vi "校准设置页.vi"() -> ()   [LabVIEW 2016, in "斯坦道CODMn新电路板.lvlib"]
uses:
  <vilib>/Analysis/6fits.llb/Curve Fitting Criteria.ctl
  <vilib>/Analysis/NI_AALPro.lvlib
  <vilib>/ptbypt/NI_PtbyPt.lvlib
panel:
  in  "公式切换阈值滴定数(0~9999)":dbl
  out "校准状态":T1(ring)
  out "模型刷新":bool
  in  "校准按钮":T2(radio)
  in  "校准导入":bool
  in  "曲线模型":T3={"标液浓度1"=0.0, "测量吸光度1"=0.0, "样品1启用"=FALSE, "标液浓度2"=0.0, "测量吸光度2"=0.0, "样品2启用"=FALSE, "标液浓度3"=0.0, "测量吸光度3"=0.0, "样品3启用"=FALSE, "标液浓度4"=0.0, "测量吸光度4"=0.0, "样品4启用"=FALSE, "标液浓度5"=0.0, "测量吸光度5"=0.0, "样品5启用"=FALSE, "模型"=enum."线性", "精度"=4.0, "XY图"=[], "拟合公式"="", "r^2"=0.0, "标样一校准时间"=timestamp(0 s since 1904-01-01), "标样二校准时间"=timestamp(0 s since 1904-01-01), "标样三校准时间"=timestamp(0 s since 1904-01-01), "标样四校准时间"=timestamp(0 s since 1904-01-01), "标样五校准时间"=timestamp(0 s since 1904-01-01), "二次方程"={"x^2"=0.0, "K"=0.0, "B"=0.0}, "标定时间"=timestamp(0 s since 1904-01-01)} {"标定时间" format="%<%Y/%m/%d %H:%M:%S>T"; "标样五校准时间" format="%<%Y/%m/%d %H:%M:%S>T"; "标样四校准时间" format="%<%Y/%m/%d %H:%M:%S>T"; "标样三校准时间" format="%<%Y/%m/%d %H:%M:%S>T"; "标样二校准时间" format="%<%Y/%m/%d %H:%M:%S>T"; "标样一校准时间" format="%<%Y/%m/%d %H:%M:%S>T"; "r^2" format="%.7f"; "测量吸光度5" format="%#.6f"; "测量吸光度4" format="%#.6f"; "测量吸光度3" format="%#.6f"; "测量吸光度2" format="%#.6f"; "测量吸光度1" format="%#.6f"}
  in  "测量模式":T4(ring)
  in  "参数下拉列表":u16(ring) items=["CODMn"=21]
  in  "量程下拉列表":enum16{"低量程1", "低量程2", "高量程1", "高量程2"}(ring)
  # "校准时间"
  # "标液浓度"
  # "滴定数"
  # "标液一"
  # "标液二"
  # "标液三"
  # "零点"
  # "跨度"
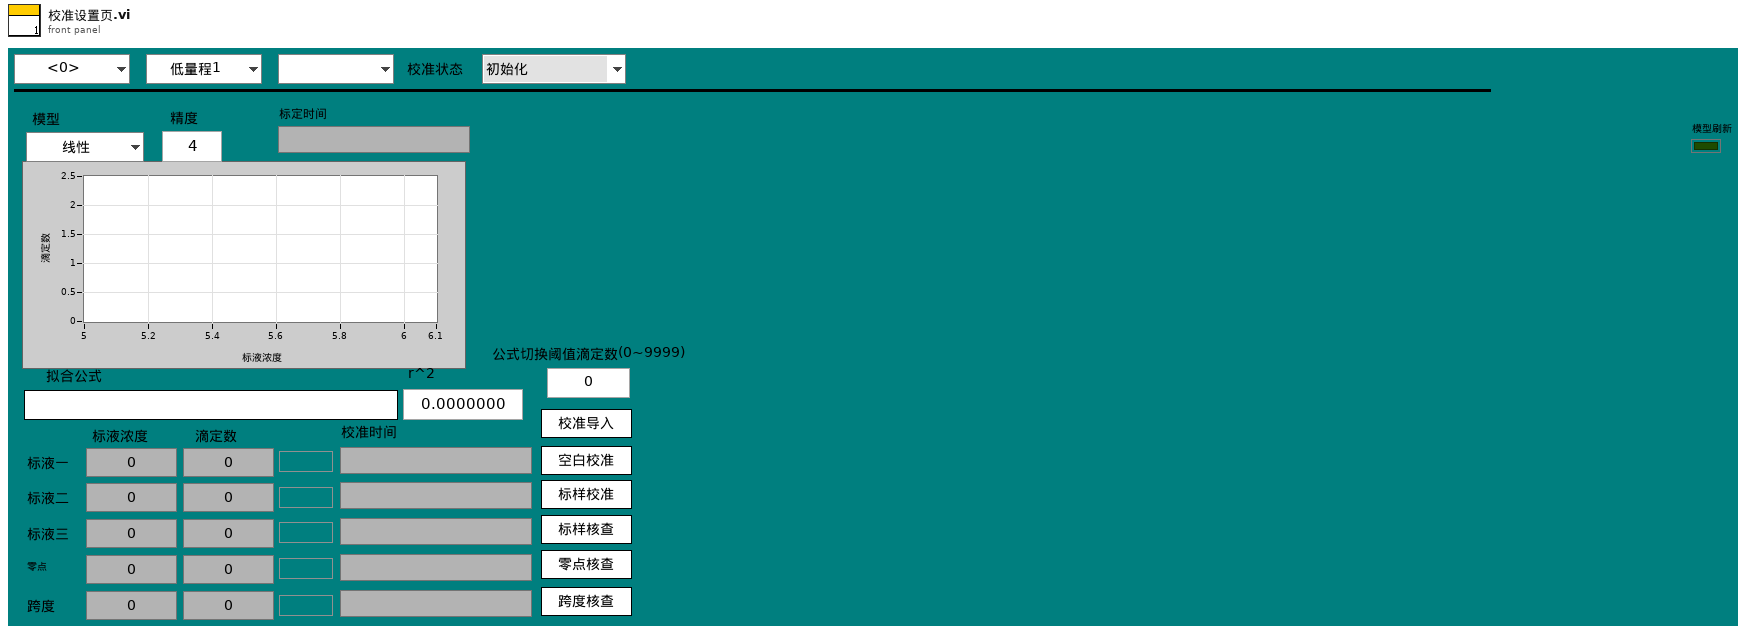
[diagram p1: front panel]
types:
  T1 = enum16{"初始化", "校准启动", "校准运行中", "测试结束", "获取校准数据", "填充校准数据", "流程结束"}
  T2 = enum32{"未选择", "空白校准", "标样校准", "标样核查", "零点核查", "跨度核查"}
  T3 = cluster{"标液浓度1":dbl, "测量吸光度1":dbl, "样品1启用":bool, "标液浓度2":dbl, "测量吸光度2":dbl, "样品2启用":bool, "标液浓度3":dbl, "测量吸光度3":dbl, "样品3启用":bool, "标液浓度4":dbl, "测量吸光度4":dbl, "样品4启用":bool, "标液浓度5":dbl, "测量吸光度5":dbl, "样品5启用":bool, "模型":enum32{"线性", "多项式"}, "精度":dbl, "XY图":cluster{"X Values":dbl[], "Y Values":dbl[]}[], "拟合公式":string, "r^2":dbl, "标样一校准时间":timestamp, "标样二校准时间":timestamp, "标样三校准时间":timestamp, "标样四校准时间":timestamp, "标样五校准时间":timestamp, "二次方程":cluster{"x^2":dbl, "K":dbl, "B":dbl}, "标定时间":timestamp}
  T4 = enum16{"", "水样测量", "标样核查", "零点核查", "跨度核查", "空白测试", "平行样测试", "加标回收"}
  T5 = enum8{"Enabled", "Disabled", "Disabled and Grayed Out"}
  T6 = cluster{"标液浓度1":dbl, "测量吸光度1":dbl, "样品1启用":bool, "标液浓度2":dbl, "测量吸光度2":dbl, "样品2启用":bool, "标液浓度3":dbl, "测量吸光度3":dbl, "样品3启用":bool, "标液浓度4":dbl, "测量吸光度4":dbl, "样品4启用":bool, "标液浓度5":dbl, "测量吸光度5":dbl, "样品5启用":bool, "模型":enum32{"线性", "多项式"}, "精度":dbl, "XY图":cluster{"X Values":dbl[], "Y Values":dbl[]}[], "拟合公式":string, "r^2":dbl, "标样一校准时间":timestamp, "标样二校准时间":timestamp, "标样三校准时间":timestamp, "标样四校准时间":timestamp, "标样五校准时间":timestamp, "二次方程":cluster{"c":dbl, "x":dbl, "x^2":dbl}, "标定时间":timestamp}[][]
  T7 = cluster{"标液浓度1":dbl, "测量吸光度1":dbl, "样品1启用":bool, "标液浓度2":dbl, "测量吸光度2":dbl, "样品2启用":bool, "标液浓度3":dbl, "测量吸光度3":dbl, "样品3启用":bool, "标液浓度4":dbl, "测量吸光度4":dbl, "样品4启用":bool, "标液浓度5":dbl, "测量吸光度5":dbl, "样品5启用":bool, "模型":enum32{"线性", "多项式"}, "精度":dbl, "XY图":cluster{"X Values":dbl[], "Y Values":dbl[]}[], "拟合公式":string, "r^2":dbl, "标样一校准时间":timestamp, "标样二校准时间":timestamp, "标样三校准时间":timestamp, "标样四校准时间":timestamp, "标样五校准时间":timestamp, "二次方程":cluster{"c":dbl, "x":dbl, "x^2":dbl}, "标定时间":timestamp}
  T8 = typedef "NI_AALPro.lvlib/Curve Fitting Criteria.ctl" = u16
  T9 = enum32{"Bad", "Idle", "Run top level", "Running"}
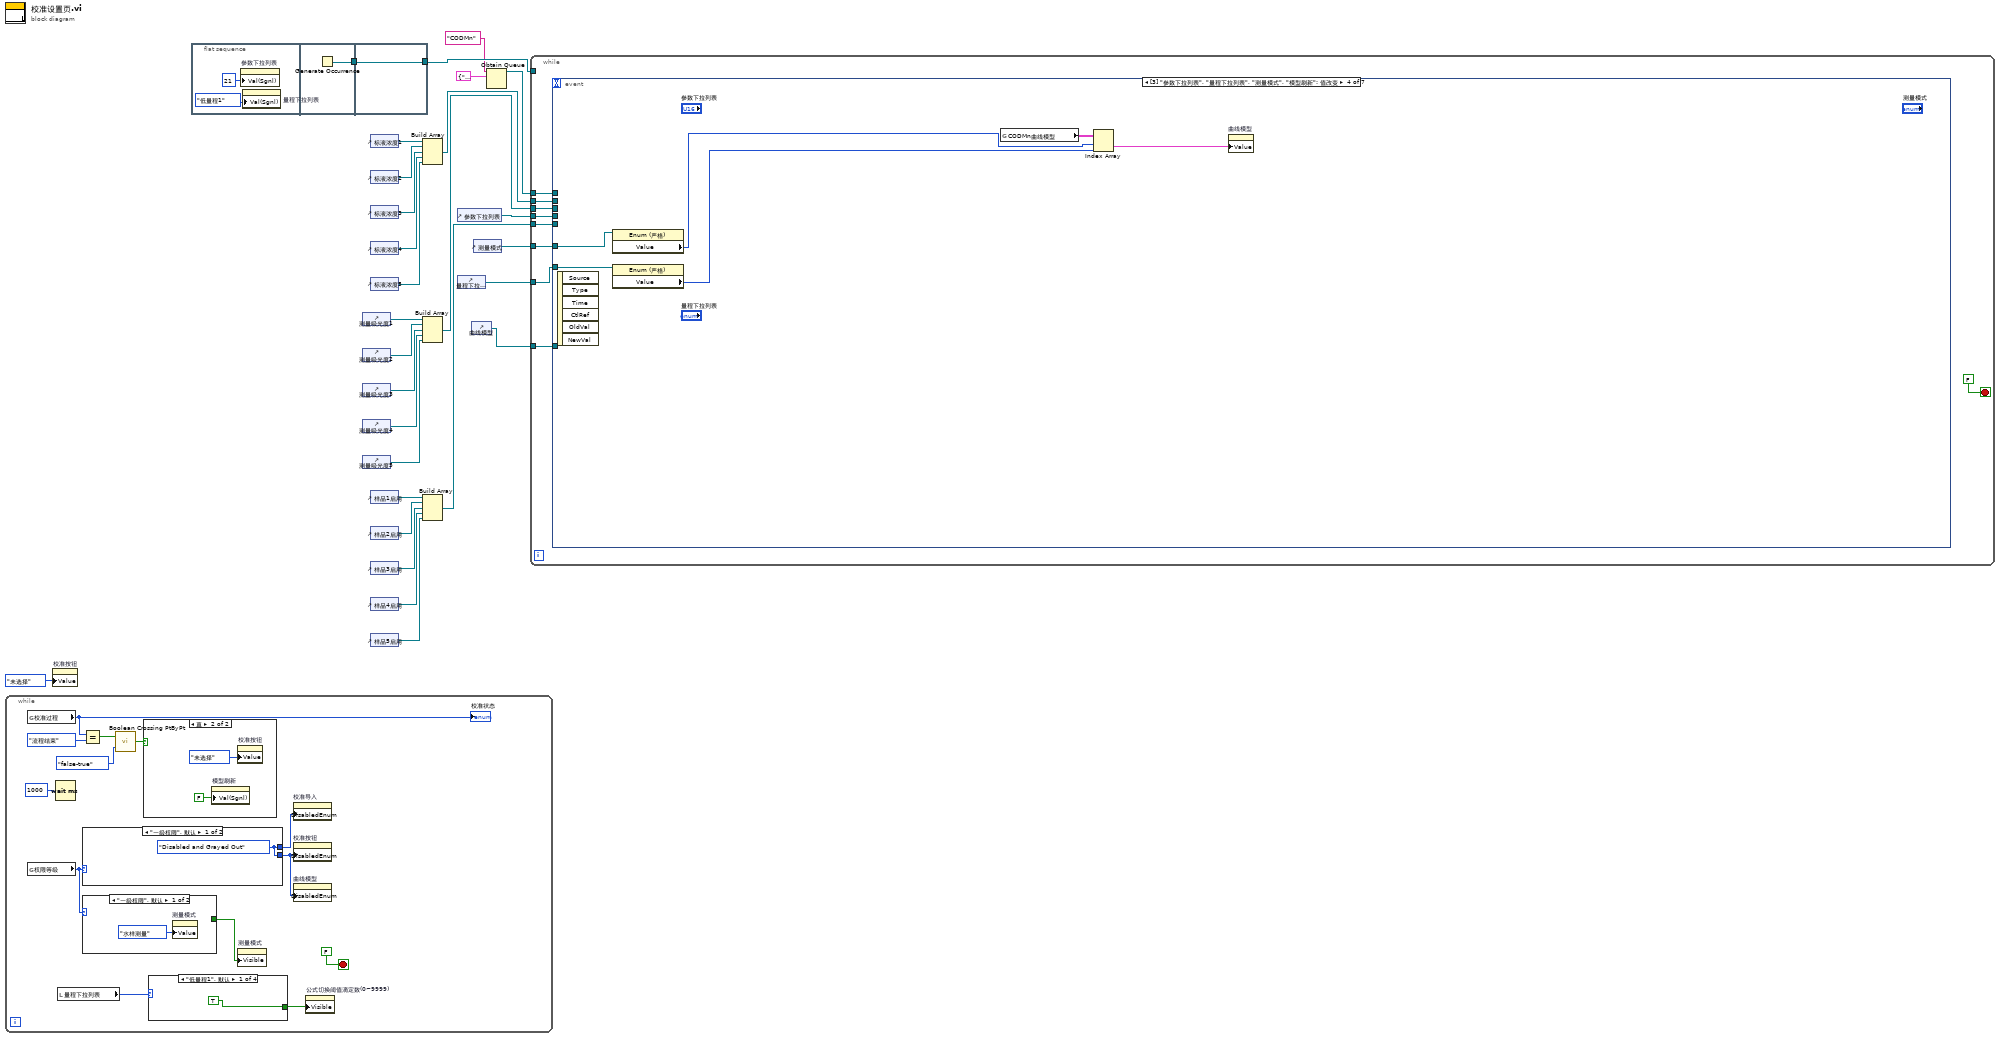
[diagram p0: block diagram]
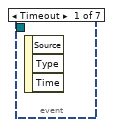
[diagram p2: hidden frame]
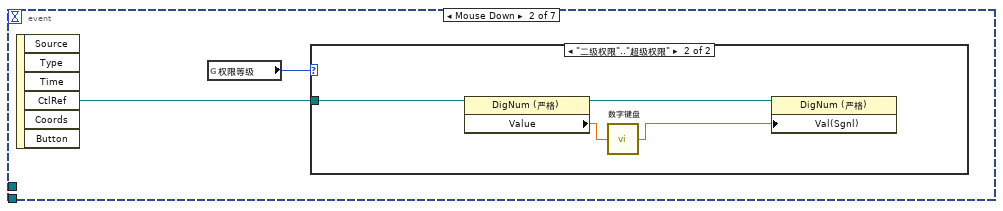
[diagram p3: hidden frame]
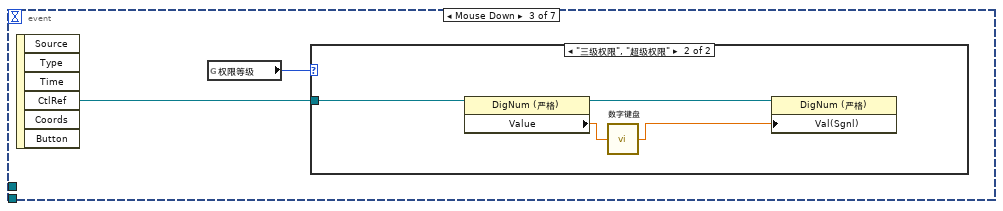
[diagram p5: hidden frame]
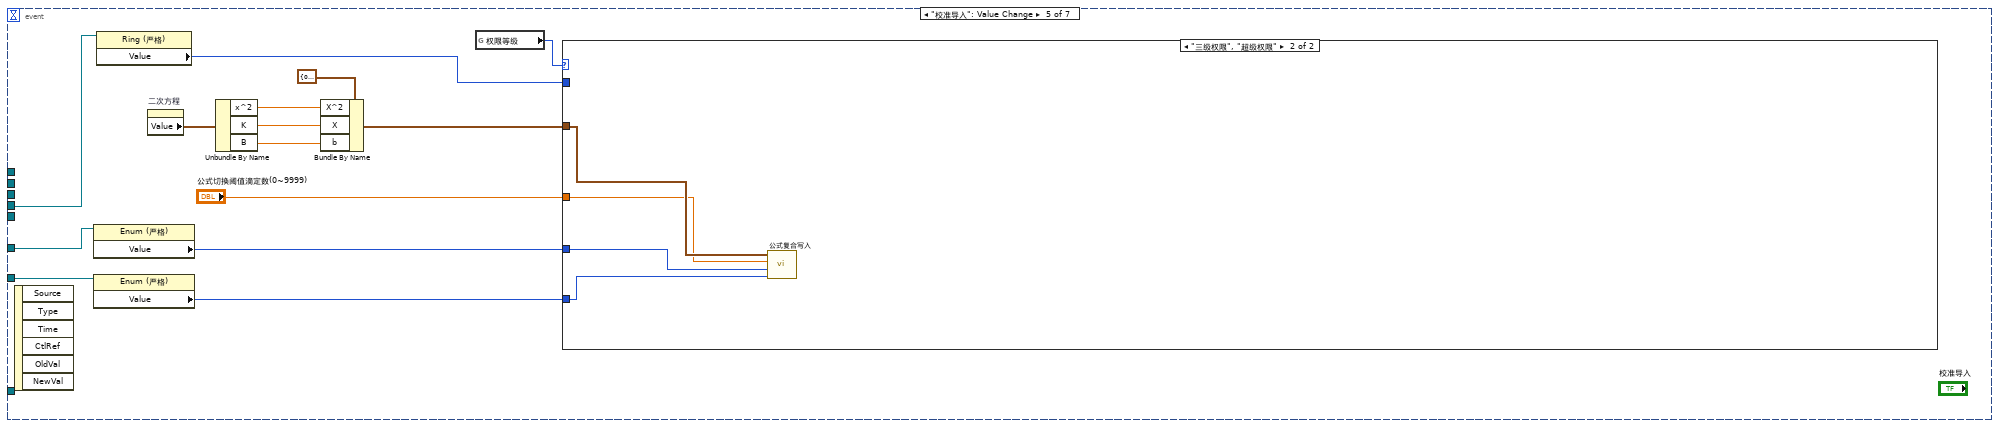
[diagram p7: hidden frame]
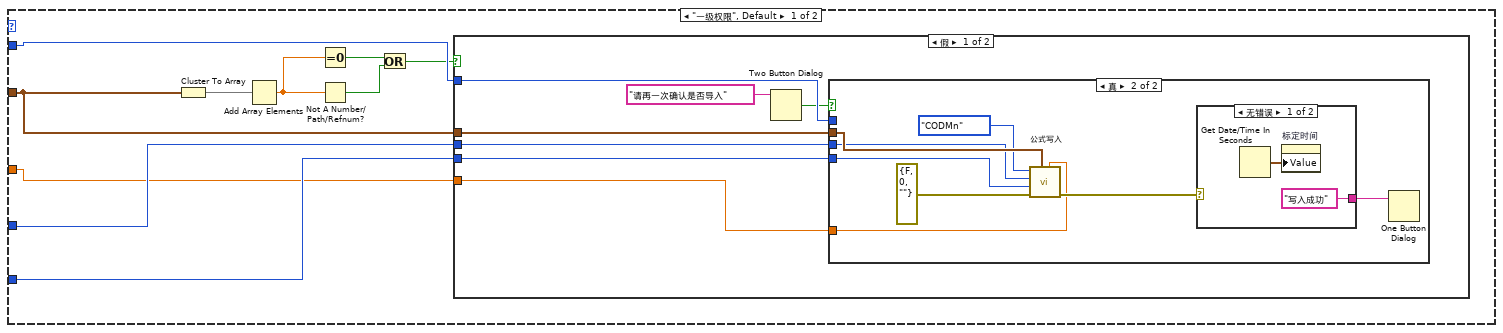
[diagram p8: hidden frame]
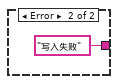
[diagram p10: hidden frame]
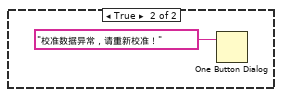
[diagram p11: hidden frame]
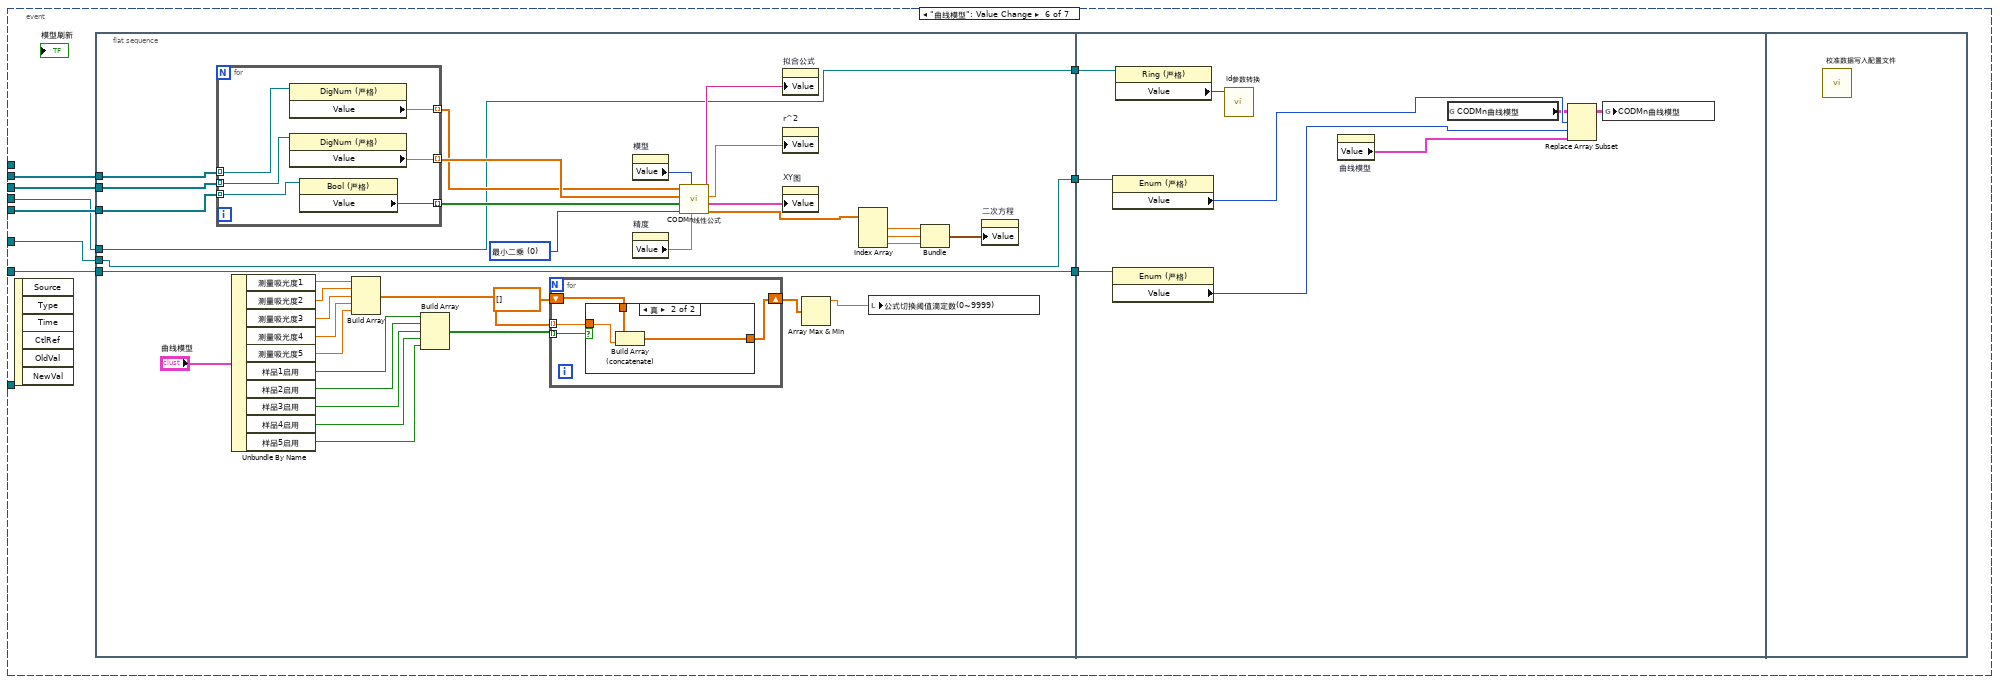
[diagram p12: hidden frame]
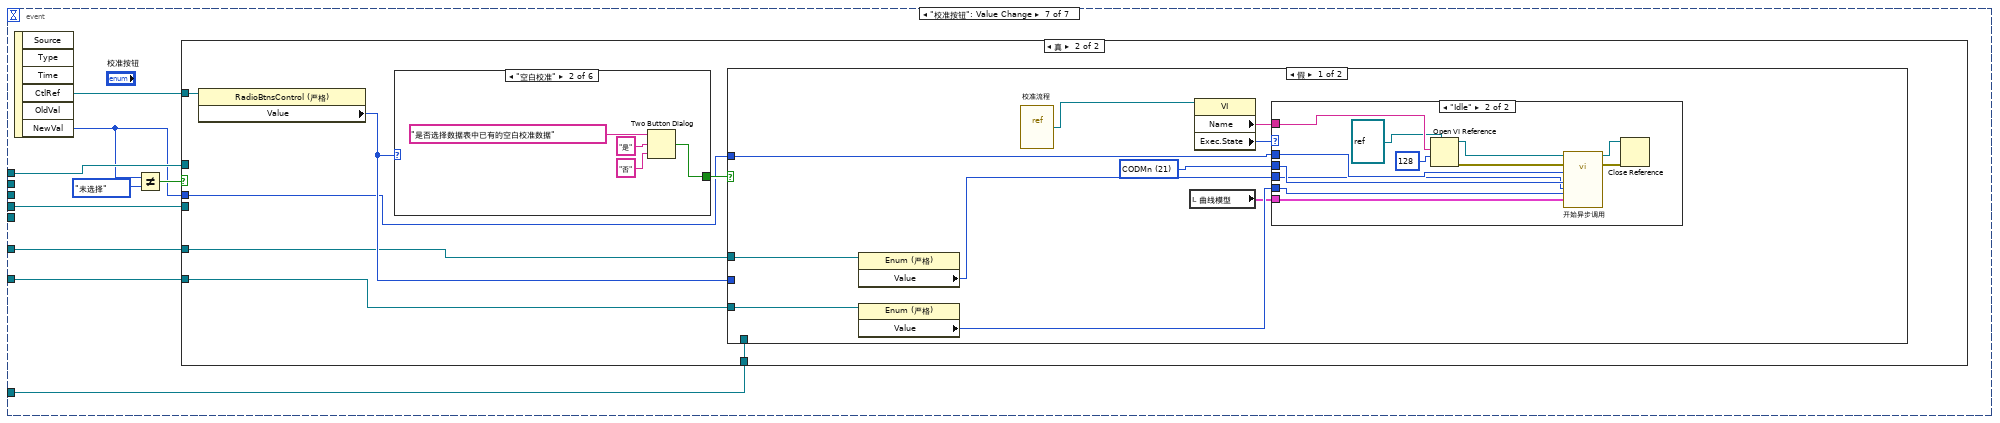
[diagram p14: hidden frame]
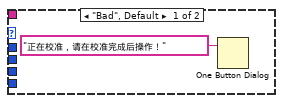
[diagram p16: hidden frame]
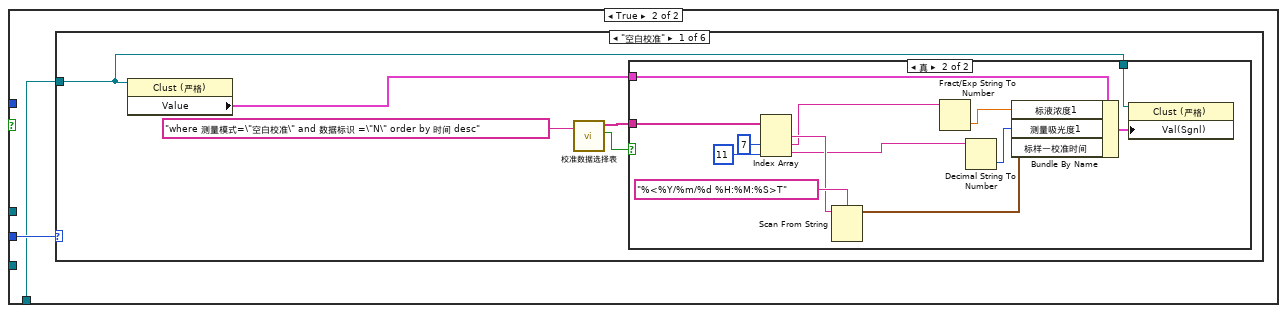
[diagram p17: hidden frame]
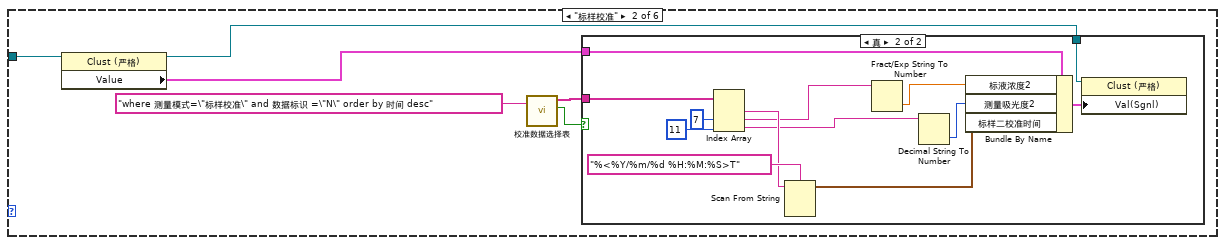
[diagram p19: hidden frame]
diagram:
  n1 = while {
    stop <- FALSE stop-if-true
    n2 = global read "VARCODMn全局变量.vi" "校准过程"() -> (w31:T1)
    "校准状态" <- w31
    n3 = global read "VARCODMn全局变量.vi" "权限等级"() -> (w38:enum16{"一级权限", "二级权限", "三级权限", "超级权限"})
    n4 = Wait (ms)(milliseconds to wait=u32 1000 ("等待时间（毫秒）")) -> ()  [unwired: 1 out]
    n5 = local read "量程下拉列表"() -> (w30:enum16{"低量程1", "低量程2", "高量程1", "高量程2"})
    n6 = case shown="\"一级权限\", 默认" w38 {
      tunnel: [w48 w49] -> w36
      tunnel: [w48 w49] -> w39
      frame "一级权限", Default {
        w48 = T5."Disabled and Grayed Out" ("禁用")
      }
      frame "二级权限".."超级权限" {
        w49 = T5."Enabled" ("禁用")
      }
    }
    n7 = case shown="\"一级权限\", 默认" w38 {
      tunnel: [_ TRUE ("可见")] -> w37
      frame "一级权限", Default {
        n8 = property on="测量模式" class="Enum (严格)"("Value"=T4."水样测量" ("测量模式")) -> ()  [unwired: 2 in, 2 out]
      }
      frame "三级权限", "超级权限" {
      }
    }
    n9 = Equal?(x=w31, y=T1."流程结束") -> (x = y?=w34:bool)
    n10 = call <vilib>:"Boolean Crossing PtByPt.vi"("direction"=enum16{"either", "false-true", "true-false"}."false-true", "input"=w34) -> ("crossing"=w32:bool)  [unwired: 1 in]
    n11 = case shown="真" w32 {
      frame False {
      }
      frame True {
        n12 = property on="模型刷新" class="Bool (严格)"("Val(Sgnl)"=FALSE ("值(信号)")) -> ()  [unwired: 2 in, 2 out]
        n13 = property on="校准按钮" class="RadioBtnsControl (严格)"("Value"=T2."未选择" ("校准按钮")) -> ()  [unwired: 2 in, 2 out]
      }
    }
    n14 = case shown="\"低量程1\", 默认" w30 {
      tunnel: [TRUE _ TRUE _] -> w29
      frame "低量程1", Default {
      }
      frame "低量程2" {
      }
      frame "高量程1" {
      }
      frame "高量程2" {
      }
    }
    n15 = property on="测量模式" class="Enum (严格)"("Visible"=w37) -> ()  [unwired: 2 in, 2 out]
    n16 = property on="校准导入" class="Bool"("DisabledEnum"=w39) -> ()  [unwired: 2 in, 2 out]
    n17 = property on="校准按钮" class="RadioBtnsControl (严格)"("DisabledEnum"=w36) -> ()  [unwired: 2 in, 2 out]
    n18 = property on="曲线模型" class="Clust (严格)"("DisabledEnum"=w36) -> ()  [unwired: 2 in, 2 out]
    n19 = property on="公式切换阈值滴定数(0~9999)" class="DigNum (严格)"("Visible"=w29) -> ()  [unwired: 2 in, 2 out]
  }
  n20 = property on="校准按钮" class="RadioBtnsControl (严格)"("Value"=T2."未选择" ("校准按钮")) -> ()  [unwired: 2 in, 2 out]
  n21 = flat-sequence {
    tunnel: [w52] -> w28
    tunnel: [w53] -> w27
    tunnel: w28 -> [w53]
    frame #0 {
      n22 = property on="参数下拉列表" class="Ring (严格)"("Val(Sgnl)"=u16 21 ("值(信号)")) -> ()  [unwired: 2 in, 2 out]
      n23 = property on="量程下拉列表" class="Enum (严格)"("Val(Sgnl)"=enum16{"低量程1", "低量程2", "高量程1", "高量程2"}."低量程1" ("值(信号)")) -> ()  [unwired: 2 in, 2 out]
    }
    frame #1 {
      n24 = Generate Occurrence() -> (w52:refnum<k4>)
    }
    frame #2 {
    }
  }
  n25 = control-ref of="测量吸光度1"() -> (w15:refnum<vi>)
  n26 = control-ref of="测量吸光度2"() -> (w16:refnum<vi>)
  n27 = control-ref of="测量吸光度3"() -> (w17:refnum<vi>)
  n28 = control-ref of="测量吸光度4"() -> (w18:refnum<vi>)
  n29 = control-ref of="测量吸光度5"() -> (w19:refnum<vi>)
  n30 = control-ref of="标液浓度1"() -> (w13:refnum<vi>)
  n31 = control-ref of="标液浓度2"() -> (w12:refnum<vi>)
  n32 = control-ref of="标液浓度3"() -> (w11:refnum<vi>)
  n33 = control-ref of="标液浓度4"() -> (w10:refnum<vi>)
  n34 = control-ref of="标液浓度5"() -> (w9:refnum<vi>)
  n35 = control-ref of="样品1启用"() -> (w25:refnum<vi>)
  n36 = control-ref of="样品2启用"() -> (w24:refnum<vi>)
  n37 = control-ref of="样品3启用"() -> (w23:refnum<vi>)
  n38 = control-ref of="样品4启用"() -> (w22:refnum<vi>)
  n39 = control-ref of="样品5启用"() -> (w21:refnum<vi>)
  n40 = Build Array(w13, w12, w11, w10, w9) -> (w8:refnum<vi>[])
  n41 = Build Array(w15, w16, w17, w18, w19) -> (w14:refnum<vi>[])
  n42 = Build Array(w25, w24, w23, w22, w21) -> (w20:refnum<vi>[])
  n43 = control-ref of="参数下拉列表"() -> (w26:refnum<vi>)
  n44 = control-ref of="量程下拉列表"() -> (w6:refnum<vi>)
  n45 = control-ref of="曲线模型"() -> (w1:refnum<vi>)
  n46 = control-ref of="测量模式"() -> (w7:refnum<vi>)
  n47 = Obtain Queue(name (unnamed)="CODMn" ("名称（未命名）"), element data type=cluster{"命令":string, "data":variant} {"命令"="", "data"=variant}) -> (queue out=w4:refnum<queue>)  [unwired: 3 in, 2 out]
  n48 = while {
    tunnel: w27 -> [_]
    tunnel: w26 -> [w61]
    tunnel: w20 -> [w60]
    tunnel: w14 -> [w59]
    tunnel: w8 -> [w58]
    tunnel: w7 -> [w57]
    tunnel: w6 -> [w56]
    tunnel: w4 -> [w55]
    tunnel: w1 -> [w54]
    stop <- FALSE stop-if-true
    n49 = event shown="[3] \"参数下拉列表\", \"量程下拉列表\", \"测量模式\", \"模型刷新\": 值改变" {
      selector: _ -> [_ _ _ _ _ _ _]
      dyn-events: _ -> [_ _ _ _ _ _ _]
      timeout: _ -> [_ _ _ _ _ _ _]
      tunnel: w61 -> [_ _ _ _ w94 w132 w203]
      tunnel: w60 -> [_ _ _ _ _ w136 _]
      tunnel: w59 -> [_ _ _ _ _ w135 _]
      tunnel: w58 -> [_ _ _ _ _ w134 _]
      tunnel: w57 -> [_ _ _ w80 w92 w130 w198]
      tunnel: w56 -> [_ _ _ w79 w90 w128 w202]
      tunnel: w55 -> [_ _ _ _ _ _ w204]
      tunnel: w54 -> [_ _ _ _ _ _ w196]
      event Timeout {
        n50 = event-data() -> ()  [unwired: 1 in, 3 out]
      }
      event "曲线模型.标液浓度1", "曲线模型.标液浓度2", "曲线模型.标液浓度3", "曲线模型.标液浓度4", "曲线模型.标液浓度5", "曲线模型.精度": Mouse Down {
        n51 = event-data() -> ("CtlRef"=w64:refnum<vi>)  [unwired: 1 in, 5 out]
        n52 = global read "VARCODMn全局变量.vi" "权限等级"() -> (w63:enum16{"一级权限", "二级权限", "三级权限", "超级权限"})
        n53 = case shown="\"二级权限\"..\"超级权限\"" w63 {
          tunnel: w64 -> [_ w68]
          frame "一级权限", Default {
          }
          frame "二级权限".."超级权限" {
            n54 = property class="DigNum (严格)"(reference=w68) -> (reference out=w66:refnum<vi>, "Value"=w67:dbl)  [unwired: 1 in, 1 out]
            n55 = call "数字键盘.vi"("OldNumber"=w67) -> ("NewNumber"=w65:dbl)
            n56 = property class="DigNum (严格)"(reference=w66, "Val(Sgnl)"=w65) -> ()  [unwired: 1 in, 2 out]
          }
        }
      }
      event "曲线模型.测量吸光度1", "曲线模型.测量吸光度2", "曲线模型.测量吸光度3", "曲线模型.测量吸光度4", "曲线模型.测量吸光度5": Mouse Down {
        n57 = event-data() -> ("CtlRef"=w70:refnum<vi>)  [unwired: 1 in, 5 out]
        n58 = global read "VARCODMn全局变量.vi" "权限等级"() -> (w69:enum16{"一级权限", "二级权限", "三级权限", "超级权限"})
        n59 = case shown="\"三级权限\", \"超级权限\"" w69 {
          tunnel: w70 -> [_ w74]
          frame "一级权限", Default {
          }
          frame "三级权限", "超级权限" {
            n60 = property class="DigNum (严格)"(reference=w74) -> (reference out=w72:refnum<vi>, "Value"=w73:dbl)  [unwired: 1 in, 1 out]
            n61 = call "数字键盘.vi"("OldNumber"=w73) -> ("NewNumber"=w71:dbl)
            n62 = property class="DigNum (严格)"(reference=w72, "Val(Sgnl)"=w71) -> ()  [unwired: 1 in, 2 out]
          }
        }
      }
      event "参数下拉列表", "量程下拉列表", "测量模式", "模型刷新": Value Change {
        n63 = event-data() -> ()  [unwired: 1 in, 6 out]
        n64 = property class="Enum (严格)"(reference=w80) -> ("Value"=w76:T4)  [unwired: 1 in, 2 out]
        n65 = property class="Enum (严格)"(reference=w79) -> ("Value"=w75:enum16{"低量程1", "低量程2", "高量程1", "高量程2"})  [unwired: 1 in, 2 out]
        n66 = global read "校准数据全局变量.vi" "CODMn曲线模型"() -> (w77:T6)
        n67 = Index Array(array=w77, index (row)=w76, index (col)=w75) -> (element=w78:T7)
        n68 = property on="曲线模型" class="Clust (严格)"("Value"=w78) -> ()  [unwired: 2 in, 2 out]
      }
      event "校准导入": Value Change {
        n69 = event-data() -> ()  [unwired: 1 in, 6 out]
        n70 = property class="Enum (严格)"(reference=w92) -> ("Value"=w91:T4)  [unwired: 1 in, 2 out]
        n71 = property class="Enum (严格)"(reference=w90) -> ("Value"=w89:enum16{"低量程1", "低量程2", "高量程1", "高量程2"})  [unwired: 1 in, 2 out]
        n72 = property class="Ring (严格)"(reference=w94) -> ("Value"=w93:u16)  [unwired: 1 in, 2 out]
        n73 = property on="二次方程" class="Clust (严格)"() -> ("Value"=w84:cluster{"x^2":dbl, "K":dbl, "B":dbl})  [unwired: 2 in, 2 out]
        n74 = Unbundle By Name(w84) -> ("x^2"=w85:dbl, "K"=w86:dbl, "B"=w87:dbl)
        n75 = Bundle By Name(cluster=cluster{"X^2":dbl, "X":dbl, "b":dbl} {"X^2"=0.0, "X"=0.0, "b"=0.0} ("公式"), "X^2"=w85, "X"=w86, "b"=w87) -> (w83:cluster{"X^2":dbl, "X":dbl, "b":dbl})
        n76 = global read "VARCODMn全局变量.vi" "权限等级"() -> (w88:enum16{"一级权限", "二级权限", "三级权限", "超级权限"})
        n77 = case shown="\"三级权限\", \"超级权限\"" w88 {
          tunnel: w93 -> [w104 _]
          tunnel: w91 -> [w103 w125]
          tunnel: w89 -> [w102 w124]
          tunnel: w83 -> [w96 w127]
          tunnel: "公式切换阈值滴定数(0~9999)" -> [w95 w126]
          frame "一级权限", Default {
            n78 = Cluster To Array(cluster=w96) -> (array=w101:dbl[])
            n79 = Add Array Elements(numeric array=w101) -> (sum=w100:dbl)
            n80 = Equal To 0?(x=w100) -> (x = 0?=w98:bool)
            n81 = Not A Number/Path/Refnum?(number/path/refnum=w100) -> (NaN/Path/Refnum?=w99:bool)
            n82 = Or(x=w98, y=w99) -> (x .or. y?=w97:bool)
            n83 = case shown="假" w97 {
              tunnel: w104 -> [w111 _]
              tunnel: w103 -> [w110 _]
              tunnel: w102 -> [w109 _]
              tunnel: w96 -> [w106 _]
              tunnel: w95 -> [w105 _]
              frame False {
                n84 = Two Button Dialog(message="请再一次确认是否导入" ("消息")) -> (T button?=w107:bool)  [unwired: 2 in]
                n85 = case shown="真" w107 {
                  tunnel: w111 -> [_ _]
                  tunnel: w110 -> [_ w113]
                  tunnel: w109 -> [_ w119]
                  tunnel: w106 -> [_ w115]
                  tunnel: w105 -> [_ w114]
                  frame False {
                  }
                  frame True {
                    n86 = call "公式写入.vi"("临界滴定数"=w114, "公式"=w115, "error in (no error)"=errorcluster {"status"=FALSE, "code"=0, "source"=""} ("error out"), "量程"=w119, "测量模式"=w113, "测量参数"=enum16{"CODMn"}."CODMn") -> ("error out"=w117:errorcluster)  [unwired: 5 in]
                    n87 = case shown="无错误" w117 {
                      tunnel: ["写入成功" "写入失败"] -> w118
                      frame No Error {
                        n88 = Get Date/Time In Seconds() -> (seconds since 1Jan1904=w120:timestamp)
                        n89 = property on="标定时间" class="AbsTime (严格)"("Value"=w120) -> ()  [unwired: 2 in, 2 out]
                      }
                      frame Error {
                      }
                    }
                    n90 = One Button Dialog(message=w118) -> ()  [unwired: 1 in, 1 out]
                  }
                }
              }
              frame True {
                n91 = One Button Dialog(message="校准数据异常，请重新校准！" ("消息")) -> ()  [unwired: 1 in, 1 out]
              }
            }
          }
          frame "三级权限", "超级权限" {
            n92 = call "公式复合写入.vi"("量程下拉列表"=w124, "测量模式"=w125, "临界滴定数"=w126, "公式"=w127) -> ()  [unwired: 8 in]
          }
        }
      }
      event "曲线模型": Value Change {
        n93 = event-data() -> ()  [unwired: 1 in, 6 out]
        n94 = flat-sequence {
          tunnel: w136 -> [w172]
          tunnel: w135 -> [w170]
          tunnel: w134 -> [w168]
          tunnel: [w155] -> w133
          tunnel: w132 -> [w155]
          tunnel: [w154] -> w131
          tunnel: w130 -> [w154]
          tunnel: [w153] -> w129
          tunnel: w128 -> [w153]
          tunnel: w133 -> [w195]
          tunnel: w131 -> [w192]
          tunnel: w129 -> [w191]
          frame #0 {
            w164 = T8 0 items=["最小二乘", "最小绝对残差", "Bisquare"] ("method")
            n95 = for {
              tunnel: w172 -> [w186] mode=indexing
              tunnel: [w185] -> w171 mode=indexing
              tunnel: w170 -> [w184] mode=indexing
              tunnel: [w183] -> w169 mode=indexing
              tunnel: w168 -> [w182] mode=indexing
              tunnel: [w181] -> w167 mode=indexing
              n96 = property class="DigNum (严格)"(reference=w182) -> ("Value"=w181:dbl)  [unwired: 1 in, 2 out]
              n97 = property class="DigNum (严格)"(reference=w184) -> ("Value"=w183:dbl)  [unwired: 1 in, 2 out]
              n98 = property class="Bool (严格)"(reference=w186) -> ("Value"=w185:bool)  [unwired: 1 in, 2 out]
            }
            n99 = Unbundle By Name("曲线模型") -> ("测量吸光度1"=w149:dbl, "测量吸光度2"=w148:dbl, "测量吸光度3"=w147:dbl, "测量吸光度4"=w145:dbl, "测量吸光度5"=w146:dbl, "样品1启用"=w144:bool, "样品2启用"=w143:bool, "样品3启用"=w142:bool, "样品4启用"=w141:bool, "样品5启用"=w140:bool)
            n100 = Build Array(w149, w148, w147, w145, w146) -> (w138:dbl[])
            n101 = Build Array(w144, w143, w142, w141, w140) -> (w139:bool[])
            n102 = for {
              tunnel: w139 -> [w176] mode=indexing
              tunnel: w138 -> [w175] mode=indexing
              shift-right: [w173] -> w151
              shift-left: dbl[] [] -> [w174]
              n103 = case shown="真" w176 {
                tunnel: w175 -> [_ w180]
                tunnel: w174 -> [w177 w179]
                tunnel: [w177 w178] -> w173
                frame False {
                }
                frame True {
                  n104 = Build Array (concatenate)(w179, w180) -> (w178:dbl[])
                }
              }
            }
            n105 = property on="模型" class="Enum (严格)"() -> ("Value"=w166:enum32{"线性", "多项式"})  [unwired: 2 in, 2 out]
            n106 = property on="精度" class="DigNum (严格)"() -> ("Value"=w165:dbl)  [unwired: 2 in, 2 out]
            n107 = call "CODMn线性公式.vi"("精度"=w165, "模型"=w166, "method"=w164, "启用"=w171, "监测浓度"=w169, "标液浓度"=w167) -> ("Polynomial Coefficients"=w160:dbl[], "XY图"=w161:cluster{"X Values":dbl[], "Y Values":dbl[]}[], "r^2"=w162:dbl, "拟合方程"=w163:string)  [unwired: 2 in]
            n108 = property on="拟合公式" class="Str"("Value"=w163) -> ()  [unwired: 2 in, 2 out]
            n109 = property on="r^2" class="DigNum (严格)"("Value"=w162) -> ()  [unwired: 2 in, 2 out]
            n110 = property on="XY图" class="XYGraph (严格)"("Value"=w161) -> ()  [unwired: 2 in, 2 out]
            n111 = Array Max & Min(array=w151) -> (max value=w137:dbl)  [unwired: 3 out]
            n112 = Index Array(array=w160) -> (element #1=w159:dbl, element #2=w158:dbl, element #3=w157:dbl)  [unwired: 3 in]
            n113 = local write "公式切换阈值滴定数(0~9999)"(w137) -> ()
            n114 = Bundle("数值"=w159, "数值"=w158, "数值"=w157) -> (w156:cluster{"数值":dbl, "数值":dbl, "数值":dbl})  [unwired: 1 in]
            n115 = property on="二次方程" class="Clust (严格)"("Value"=w156) -> ()  [unwired: 2 in, 2 out]
          }
          frame #1 {
            n116 = property class="Enum (严格)"(reference=w192) -> ("Value"=w189:T4)  [unwired: 1 in, 2 out]
            n117 = property class="Enum (严格)"(reference=w191) -> ("Value"=w190:enum16{"低量程1", "低量程2", "高量程1", "高量程2"})  [unwired: 1 in, 2 out]
            n118 = property class="Ring (严格)"(reference=w195) -> ("Value"=w194:u16)  [unwired: 1 in, 2 out]
            n119 = call "id参数转换.vi"("id"=w194) -> ()  [unwired: 10 in, 1 out]
            n120 = property on="曲线模型" class="Clust (严格)"() -> ("Value"=w193:T3)  [unwired: 2 in, 2 out]
            n121 = global read "校准数据全局变量.vi" "CODMn曲线模型"() -> (w188:T6)
            n122 = Replace Array Subset(array=w188, new element=w193, index (row)=w189, index (col)=w190) -> (w187:T6)
            n123 = global write "校准数据全局变量.vi" "CODMn曲线模型"(w187) -> ()
          }
          frame #2 {
            n124 = call "校准数据写入配置文件.vi"() -> ()  [unwired: 11 in, 1 out]
          }
        }
      }
      event "校准按钮": Value Change {
        n125 = event-data() -> ("CtlRef"=w197:refnum<vi>, "NewVal"=w199:T2)  [unwired: 1 in, 4 out]
        n126 = Not Equal?(x=w199, y=T2."未选择") -> (x != y?=w200:bool)
        n127 = case shown="真" w200 {
          tunnel: w204 -> [_ _]
          tunnel: w203 -> [_ _]
          tunnel: w202 -> [_ w207]
          tunnel: w199 -> [_ w208]
          tunnel: w198 -> [_ w206]
          tunnel: w197 -> [_ w211]
          tunnel: w196 -> [_ w205]
          frame False {
          }
          frame True {
            n128 = property class="RadioBtnsControl (严格)"(reference=w211) -> ("Value"=w209:T2)  [unwired: 1 in, 2 out]
            n129 = case shown="\"空白校准\"" w209 {
              tunnel: [_ w327 w331 w335 w339 w343] -> w210
              frame "未选择", Default {
              }
              frame "空白校准" {
                n130 = Two Button Dialog(message="是否选择数据表中已有的空白校准数据" ("消息"), 1:"否" ("F按钮名称（“取消”）"), 2:"是" ("T按钮名称（“确定”）")) -> (T button?=w327:bool)
              }
              frame "标样校准" {
                n131 = Two Button Dialog(message="是否选择数据表中已有的标样校准数据" ("消息"), 1:"否" ("F按钮名称（“取消”）"), 2:"是" ("T按钮名称（“确定”）")) -> (T button?=w331:bool)
              }
              frame "标样核查" {
                n132 = Two Button Dialog(message="是否选择数据表中已有的标样校准数据" ("消息"), 1:"否" ("F按钮名称（“取消”）"), 2:"是" ("T按钮名称（“确定”）")) -> (T button?=w335:bool)
              }
              frame "零点核查" {
                n133 = Two Button Dialog(message="是否选择数据表中已有的标样校准数据" ("消息"), 1:"否" ("F按钮名称（“取消”）"), 2:"是" ("T按钮名称（“确定”）")) -> (T button?=w339:bool)
              }
              frame "跨度核查" {
                n134 = Two Button Dialog(message="是否选择数据表中已有的标样校准数据" ("消息"), 1:"否" ("F按钮名称（“取消”）"), 2:"是" ("T按钮名称（“确定”）")) -> (T button?=w343:bool)
              }
            }
            n135 = case shown="假" w210 {
              tunnel: w209 -> [_ w236]
              tunnel: w205 -> [_ w235]
              tunnel: w208 -> [w216 _]
              tunnel: w207 -> [w215 _]
              tunnel: w206 -> [w213 _]
              frame False {
                w212 = u16 21 items=["CODMn"=21] ("参数下拉列表")
                n136 = property class="Enum (严格)"(reference=w213) -> ("Value"=w214:T4)  [unwired: 1 in, 2 out]
                n137 = property class="Enum (严格)"(reference=w215) -> ("Value"=w218:enum16{"低量程1", "低量程2", "高量程1", "高量程2"})  [unwired: 1 in, 2 out]
                n138 = vi-ref "校准流程.vi"() -> (w219:refnum<vi>)
                n139 = local read "曲线模型"() -> (w217:T3)
                n140 = property class="VI"(reference=w219) -> ("Name"=w220:string, "Exec.State"=w221:T9)  [unwired: 1 in, 2 out]
                n141 = case shown="\"Idle\"" w221 {
                  tunnel: w220 -> [_ w234]
                  tunnel: w216 -> [_ w227]
                  tunnel: w212 -> [_ w226]
                  tunnel: w214 -> [_ w225]
                  tunnel: w218 -> [_ w224]
                  tunnel: w217 -> [_ w223]
                  frame "Bad", Default {
                    n142 = One Button Dialog(message="正在校准，请在校准完成后操作！" ("消息")) -> ()  [unwired: 1 in, 1 out]
                  }
                  frame "Idle" {
                    n143 = Open VI Reference(type specifier VI Refnum (for type only)=refnum<vi> refnum, vi path=w234, options=128 ("选项")) -> (vi reference=w232:refnum<vi>, error out=w231:errorcluster)  [unwired: 3 in]
                    n144 = call-by-ref "开始异步调用"(reference=w232, error in=w231, "校准模式"=w227, "参数下拉列表"=w226, "测量模式"=w225, "量程下拉列表"=w224, "曲线模型"=w223) -> (reference out=w229:refnum<vi>, error out=w230:errorcluster)  [unwired: 11 in]
                    n145 = Close Reference(reference=w229, error in (no error)=w230) -> ()  [unwired: 1 out]
                  }
                }
              }
              frame True {
                n146 = case shown="\"空白校准\"" w236 {
                  tunnel: w235 -> [w241 w259 w277 w295 w313 _]
                  frame "空白校准" {
                    n147 = property class="Clust (严格)"(reference=w241) -> ("Value"=w240:T3)  [unwired: 1 in, 2 out]
                    n148 = call "校准数据选择表.vi"("condition"="where 测量模式=\"空白校准\" and 数据标识 =\"N\" order by 时间 desc") -> ("布尔"=w237:bool, "ItemNames"=w239:string[])  [unwired: 9 in]
                    n149 = case shown="真" w237 {
                      tunnel: w241 -> [_ w254]
                      tunnel: w240 -> [_ w253]
                      tunnel: w239 -> [_ w248]
                      frame False {
                      }
                      frame True {
                        n150 = Index Array(array=w248, index #2=7 ("索引"), index #3=11 ("索引")) -> (element #1=w245:string, element #2=w243:string, element #3=w244:string)  [unwired: 1 in]
                        n151 = Scan From String(format string="%<%Y/%m/%d %H:%M:%S>T" ("格式字符串"), input string=w245) -> (output 1=w250:timestamp)  [unwired: 3 in, 3 out]
                        n152 = Fract/Exp String To Number(string=w243) -> (number=w242:dbl)  [unwired: 3 in, 1 out]
                        n153 = Decimal String To Number(string=w244) -> (number=w249:i32)  [unwired: 2 in, 1 out]
                        n154 = Bundle By Name(cluster=w253, "标液浓度1"=w242, "测量吸光度1"=w249, "标样一校准时间"=w250) -> (w252:T3)
                        n155 = property class="Clust (严格)"(reference=w254, "Val(Sgnl)"=w252) -> ()  [unwired: 1 in, 2 out]
                      }
                    }
                  }
                  frame "标样校准" {
                    n156 = property class="Clust (严格)"(reference=w259) -> ("Value"=w258:T3)  [unwired: 1 in, 2 out]
                    n157 = call "校准数据选择表.vi"("condition"="where 测量模式=\"标样校准\" and 数据标识 =\"N\" order by 时间 desc") -> ("布尔"=w255:bool, "ItemNames"=w257:string[])  [unwired: 9 in]
                    n158 = case shown="真" w255 {
                      tunnel: w259 -> [_ w272]
                      tunnel: w258 -> [_ w271]
                      tunnel: w257 -> [_ w266]
                      frame False {
                      }
                      frame True {
                        n159 = Index Array(array=w266, index #2=7 ("索引"), index #3=11 ("索引")) -> (element #1=w263:string, element #2=w261:string, element #3=w262:string)  [unwired: 1 in]
                        n160 = Scan From String(format string="%<%Y/%m/%d %H:%M:%S>T" ("格式字符串"), input string=w263) -> (output 1=w268:timestamp)  [unwired: 3 in, 3 out]
                        n161 = Fract/Exp String To Number(string=w261) -> (number=w260:dbl)  [unwired: 3 in, 1 out]
                        n162 = Decimal String To Number(string=w262) -> (number=w267:i32)  [unwired: 2 in, 1 out]
                        n163 = Bundle By Name(cluster=w271, "标液浓度2"=w260, "测量吸光度2"=w267, "标样二校准时间"=w268) -> (w270:T3)
                        n164 = property class="Clust (严格)"(reference=w272, "Val(Sgnl)"=w270) -> ()  [unwired: 1 in, 2 out]
                      }
                    }
                  }
                  frame "标样核查" {
                    n165 = property class="Clust (严格)"(reference=w277) -> ("Value"=w276:T3)  [unwired: 1 in, 2 out]
                    n166 = call "校准数据选择表.vi"("condition"="where 测量模式=\"标样核查\" and 数据标识 =\"N\" order by 时间 desc") -> ("布尔"=w273:bool, "ItemNames"=w274:string[])  [unwired: 9 in]
                    n167 = case shown="真" w273 {
                      tunnel: w277 -> [_ w290]
                      tunnel: w276 -> [_ w289]
                      tunnel: w274 -> [_ w281]
                      frame False {
                      }
                      frame True {
                        n168 = Index Array(array=w281, index #2=7 ("索引"), index #3=11 ("索引")) -> (element #1=w280:string, element #2=w279:string, element #3=w278:string)  [unwired: 1 in]
                        n169 = Scan From String(format string="%<%Y/%m/%d %H:%M:%S>T" ("格式字符串"), input string=w280) -> (output 1=w286:timestamp)  [unwired: 3 in, 3 out]
                        n170 = Fract/Exp String To Number(string=w279) -> (number=w285:dbl)  [unwired: 3 in, 1 out]
                        n171 = Decimal String To Number(string=w278) -> (number=w284:i32)  [unwired: 2 in, 1 out]
                        n172 = Bundle By Name(cluster=w289, "标液浓度3"=w285, "测量吸光度3"=w284, "标样三校准时间"=w286) -> (w288:T3)
                        n173 = property class="Clust (严格)"(reference=w290, "Val(Sgnl)"=w288) -> ()  [unwired: 1 in, 2 out]
                      }
                    }
                  }
                  frame "零点核查" {
                    n174 = property class="Clust (严格)"(reference=w295) -> ("Value"=w294:T3)  [unwired: 1 in, 2 out]
                    n175 = call "校准数据选择表.vi"("condition"="where 测量模式=\"零点核查\" and 数据标识 =\"N\" order by 时间 desc") -> ("布尔"=w291:bool, "ItemNames"=w292:string[])  [unwired: 9 in]
                    n176 = case shown="真" w291 {
                      tunnel: w295 -> [_ w308]
                      tunnel: w294 -> [_ w307]
                      tunnel: w292 -> [_ w300]
                      frame False {
                      }
                      frame True {
                        n177 = Index Array(array=w300, index #2=7 ("索引"), index #3=11 ("索引")) -> (element #1=w299:string, element #2=w297:string, element #3=w298:string)  [unwired: 1 in]
                        n178 = Scan From String(format string="%<%Y/%m/%d %H:%M:%S>T" ("格式字符串"), input string=w299) -> (output 1=w304:timestamp)  [unwired: 3 in, 3 out]
                        n179 = Fract/Exp String To Number(string=w297) -> (number=w296:dbl)  [unwired: 3 in, 1 out]
                        n180 = Decimal String To Number(string=w298) -> (number=w303:i32)  [unwired: 2 in, 1 out]
                        n181 = Bundle By Name(cluster=w307, "标液浓度4"=w296, "测量吸光度4"=w303, "标样四校准时间"=w304) -> (w306:T3)
                        n182 = property class="Clust (严格)"(reference=w308, "Val(Sgnl)"=w306) -> ()  [unwired: 1 in, 2 out]
                      }
                    }
                  }
                  frame "跨度核查" {
                    n183 = property class="Clust (严格)"(reference=w313) -> ("Value"=w312:T3)  [unwired: 1 in, 2 out]
                    n184 = call "校准数据选择表.vi"("condition"="where 测量模式=\"跨度核查\" and 数据标识 =\"N\" order by 时间 desc") -> ("布尔"=w309:bool, "ItemNames"=w310:string[])  [unwired: 9 in]
                    n185 = case shown="真" w309 {
                      tunnel: w313 -> [_ w326]
                      tunnel: w312 -> [_ w325]
                      tunnel: w310 -> [_ w320]
                      frame False {
                      }
                      frame True {
                        n186 = Index Array(array=w320, index #2=7 ("索引"), index #3=11 ("索引")) -> (element #1=w319:string, element #2=w315:string, element #3=w316:string)  [unwired: 1 in]
                        n187 = Scan From String(format string="%<%Y/%m/%d %H:%M:%S>T" ("格式字符串"), input string=w319) -> (output 1=w322:timestamp)  [unwired: 3 in, 3 out]
                        n188 = Fract/Exp String To Number(string=w315) -> (number=w314:dbl)  [unwired: 3 in, 1 out]
                        n189 = Decimal String To Number(string=w316) -> (number=w321:i32)  [unwired: 2 in, 1 out]
                        n190 = Bundle By Name(cluster=w325, "标液浓度5"=w314, "测量吸光度5"=w321, "标样五校准时间"=w322) -> (w324:T3)
                        n191 = property class="Clust (严格)"(reference=w326, "Val(Sgnl)"=w324) -> ()  [unwired: 1 in, 2 out]
                      }
                    }
                  }
                  frame "未选择" {
                  }
                }
              }
            }
          }
        }
      }
    }
  }
